vi "GetVbreakStartTdmConfig.vi"(0 "storage refnum (file)":refnum<k20>, 1 "error in":errorcluster) -> (2 "storage refnum (file) out":refnum<k20>, 3 "output cluster":T1={"Range"=0.0, "Ilim"=0.0, "Level"=0.0, "Channel"=1, "Timed Totalize"=0.1} {"Channel" items=["Channel 1"=1, "Channel 2"=2]}, 4 "error out":errorcluster)   [LabVIEW 2014]
uses:
  VBreakInitialCond.ctl
  <vilib>/Platform/storage/lvStorage.llb/_queryPropPoly.vi
  <vilib>/Platform/storage/lvStorage.llb/_queryPropString.vi
  <vilib>/Platform/storage/lvStorage.llb/_queryGenericObjects.vi
  <vilib>/Platform/storage/lvStorage.llb/_loadAllDdt.vi
  <vilib>/Platform/storage/lvStorage.llb/xStorage/xStorageSupp/ErrorOut.vi
  <vilib>/Platform/storage/lvStorage.llb/xStorage/Read Data/Read Data.xnode
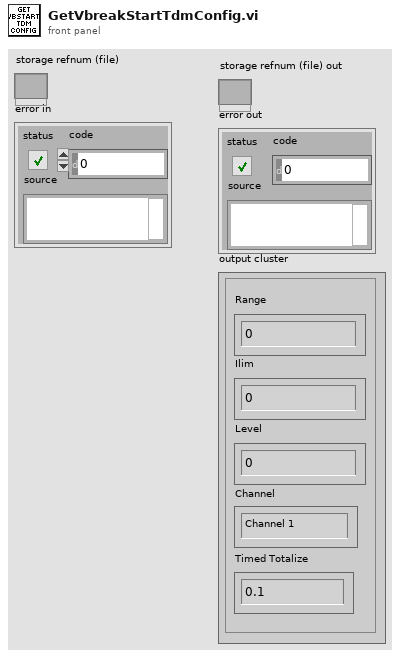
[diagram p1: front panel]
types:
  T1 = typedef "VBreakInitialCond.ctl" = cluster{"Range":dbl, "Ilim":dbl, "Level":dbl, "Channel":i32, "Timed Totalize":dbl}
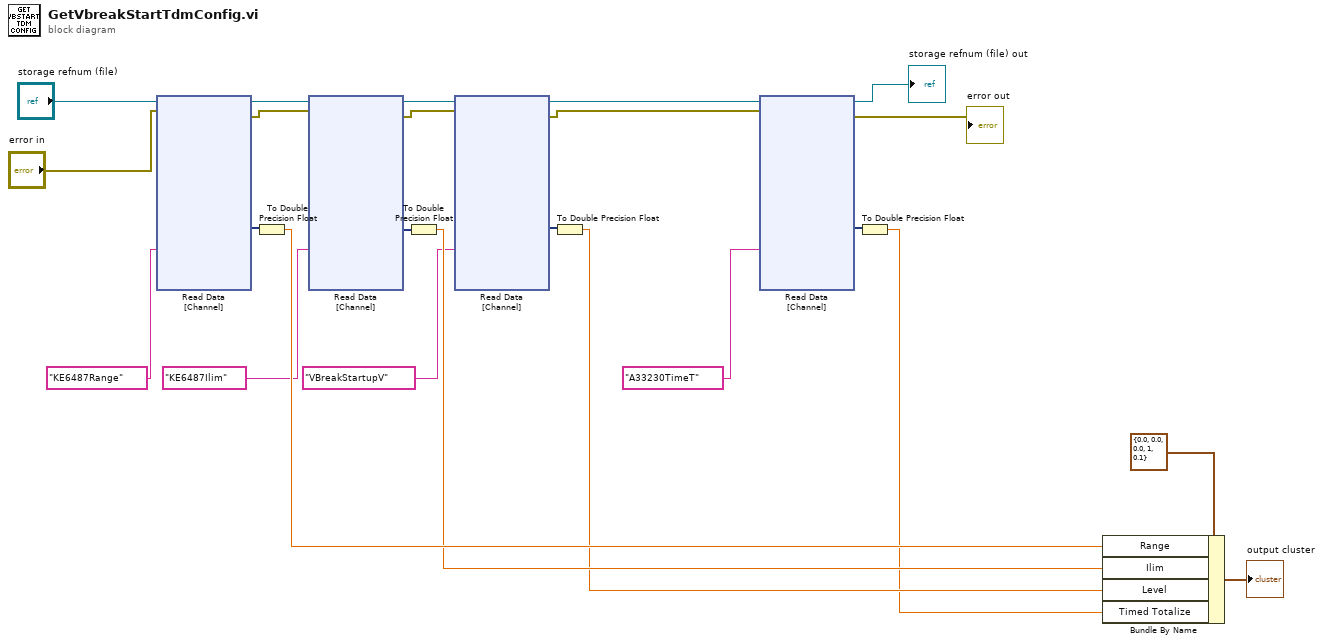
[diagram p0: block diagram]
diagram:
  n1 = xnode "Read Data\n[Channel]"("Name"="KE6487Range", "storage refnum (file)"="storage refnum (file)", "error in"="error in") -> ("Signal"=w23:dynamicdata, "storage refnum (file) out"=w19:refnum<k20>, "error out"=w17:errorcluster)  [unwired: 3 in, 1 out]
  n2 = To Double Precision Float(number=w23) -> (double precision float=w15:dbl)
  n3 = xnode "Read Data\n[Channel]"("Name"="KE6487Ilim", "storage refnum (file)"=w19, "error in"=w17) -> ("Signal"=w22:dynamicdata, "storage refnum (file) out"=w18:refnum<k20>, "error out"=w16:errorcluster)  [unwired: 3 in, 1 out]
  n4 = To Double Precision Float(number=w22) -> (double precision float=w14:dbl)
  n5 = xnode "Read Data\n[Channel]"("Name"="VBreakStartupV", "storage refnum (file)"=w18, "error in"=w16) -> ("Signal"=w21:dynamicdata, "storage refnum (file) out"=w3:refnum<k20>, "error out"=w2:errorcluster)  [unwired: 3 in, 1 out]
  n6 = To Double Precision Float(number=w21) -> (double precision float=w13:dbl)
  n7 = xnode "Read Data\n[Channel]"("Name"="A33230TimeT", "storage refnum (file)"=w3, "error in"=w2) -> ("Signal"=w20:dynamicdata, "storage refnum (file) out"=→"storage refnum (file) out":refnum<k20>, "error out"=→"error out":errorcluster)  [unwired: 3 in, 1 out]
  n8 = To Double Precision Float(number=w20) -> (double precision float=w1:dbl)
  n9 = Bundle By Name(cluster=T1 {"Range"=0.0, "Ilim"=0.0, "Level"=0.0, "Channel"=1, "Timed Totalize"=0.1} ("Condition Initial"), "Range"=w15, "Ilim"=w14, "Level"=w13, "Timed Totalize"=w1) -> (→"output cluster":T1)
